vi "TCP- Client.vi"() -> ()   [LabVIEW 2015]
doc: "Demonstrates how to use Network Streams to pass data and commands between two running VIs. This VI passes data to the host VI, based on the frequency specified by the host VI."
panel:
  out "Cluster":cluster{"Frequency":i32}={"Frequency"=10}
  in  "Stop":bool
  in  "Server Closed":string="The server VI closed the connection."
  in  "Client Closed":string="The client VI closed the connection."
  # "Overview: Demonstrates how to use Network Streams to pass data and commands between two running VIs.\nRequirements: Windows\nInstructions:\n1. Run this VI.\n2. Open Simple Network Streams - Host.vi and follow the instructions on its front panel."
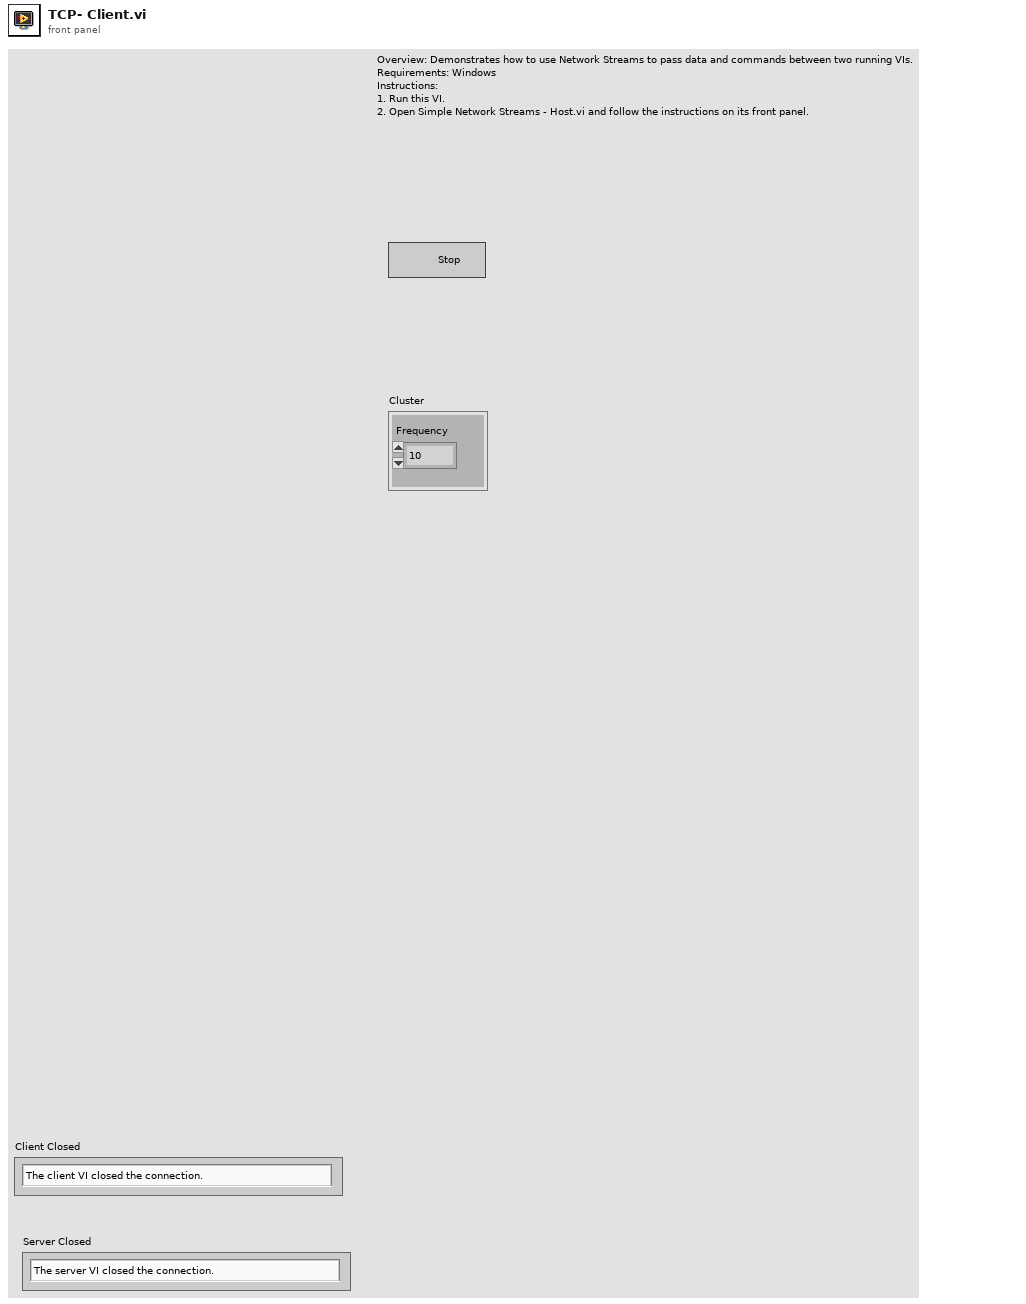
[diagram p1: front panel]
types:
  T1 = cluster{"ID":dbl, "Enable":dbl, "Direction":dbl, "Brake":dbl, "Built-In Encoder":dbl, "Motor Voltage FB":dbl, "Motor Current FB":dbl, "Brake Voltage FB":dbl, "Brake Current FB":dbl, "Up Limit Switch":dbl, "Down Limit Switch":dbl, "Up Limit Config":dbl, "Down Limit Config":dbl, "Motor Current Limit Config":dbl, "Brake Current Limit Config":dbl, "Status":dbl}
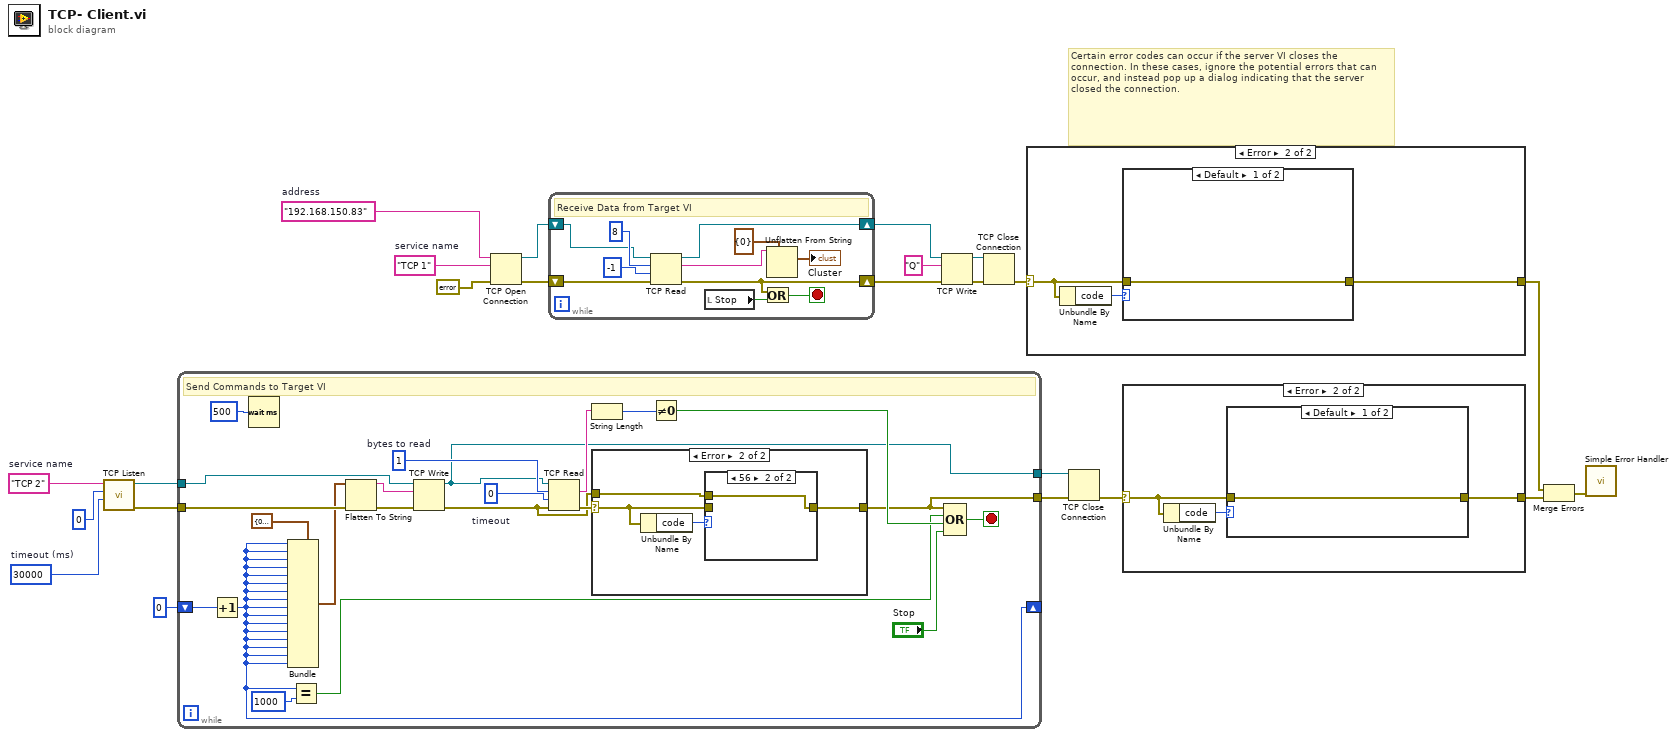
[diagram p0: block diagram]
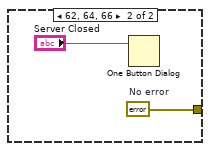
[diagram p3: hidden frame]
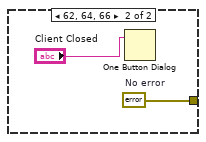
[diagram p5: hidden frame]
diagram:
  w5 = "TCP 1"  # service name
  w17 = "192.168.150.83"  # address
  w6 = "TCP 2"  # service name
  w22 = 30000  # timeout (ms)
  # "Certain error codes can occur if the server VI closes the connection. In these cases, ignore the potential errors that can occur, and instead pop up a dialog indicating that the server closed the connection."
  n1 = call <vilib>:"TCP Listen.vi"("timeout ms (wait forever: -1)"=w22, "port"=u16 0, "service name"=w6) -> ("error out"=w3:errorcluster, "connection ID"=w21:refnum<k5>)  [unwired: 4 in, 3 out]
  n2 = while "Host->Target Command Writer" {
    tunnel: w3 -> [w32]
    tunnel: w21 -> [w45]
    tunnel: [w36] -> w19
    tunnel: [w35] -> w18
    shift-right: [w26] -> _
    shift-left: 0 -> [w29]
    stop <- w38 stop-if-true
    w41 = 0  # timeout
    w40 = 1  # bytes to read
    # "Send Commands to Target VI"
    n3 = Increment(x=w29) -> (x+1=w26:i32)
    n4 = Wait (ms)(milliseconds to wait=u32 500) -> ()  [unwired: 1 out]
    n5 = Bundle(cluster=T1 {"ID"=0.0, "Enable"=0.0, "Direction"=0.0, "Brake"=0.0, "Built-In Encoder"=0.0, "Motor Voltage FB"=0.0, "Motor Current FB"=0.0, "Brake Voltage FB"=0.0, "Brake Current FB"=0.0, "Up Limit Switch"=0.0, "Down Limit Switch"=0.0, "Up Limit Config"=0.0, "Down Limit Config"=0.0, "Motor Current Limit Config"=0.0, "Brake Current Limit Config"=0.0, "Status"=0.0} ("MirrorCoverMotor"), "ID"=w26, "Enable"=w26, "Direction"=w26, "Brake"=w26, "Built-In Encoder"=w26, "Motor Voltage FB"=w26, "Motor Current FB"=w26, "Brake Voltage FB"=w26, "Brake Current FB"=w26, "Up Limit Switch"=w26, "Down Limit Switch"=w26, "Up Limit Config"=w26, "Down Limit Config"=w26, "Motor Current Limit Config"=w26, "Brake Current Limit Config"=w26, "Status"=w26) -> (w30:T1)
    n6 = Equal?(x=w26, y=1000) -> (x = y?=w27:bool)
    n7 = Flatten To String(anything=w30, error in (no error)=w32) -> (data string=w34:string, error out=w33:errorcluster)  [unwired: 2 in, 1 out]
    n8 = TCP Write(connection ID=w45, data in=w34, error in (no error)=w33) -> (connection ID out=w35:refnum<k5>, error out=w39:errorcluster)  [unwired: 2 out]
    n9 = TCP Read(connection ID=w35, bytes to read=w40, error in (no error)=w39, 9:w41) -> (data out=w43:string, error out=w44:errorcluster)  [unwired: 2 out]
    n10 = String Length(string=w43) -> (length=w42:i32)
    n11 = case shown="Error" w44 {
      selector: w44 -> [w46 w49]
      tunnel: [w46 w47] -> w36
      tunnel: w39 -> [_ w48]
      frame No Error {
      }
      frame Error {
        n12 = Unbundle By Name(w49) -> ("code"=w50:i32)
        n13 = case shown="56" w50 {
          tunnel: w49 -> [w51 _]
          tunnel: w48 -> [_ w52]
          tunnel: [w51 w52] -> w47
          frame Default {
          }
          frame 56 {
          }
        }
      }
    }
    n14 = Not Equal To 0?(x=w42) -> (x != 0?=w37:bool)
    n15 = Compound Arithmetic op=OR(w36, w27, w37, "Stop") -> (w38:bool)
  }
  n16 = TCP Open Connection(address=w17, remote port or service name=w5, error in (no error)=errorcluster {"status"=FALSE, "code"=0, "source"=""} ("error out")) -> (connection ID=w16:refnum<k5>, error out=w1:errorcluster)  [unwired: 2 in]
  n17 = while "Target->Host Data Reader" {
    shift-right: [w56] -> w11
    shift-left: w1 -> [w61]
    shift-right: [w60] -> w10
    shift-left: w16 -> [w59]
    stop <- w57 stop-if-true
    # "Receive Data from Target VI"
    n18 = TCP Read(connection ID=w59, bytes to read=8, error in (no error)=w61, 9:-1 ("timeout ms (25000)")) -> (connection ID out=w60:refnum<k5>, data out=w55:string, error out=w56:errorcluster)  [unwired: 1 in]
    n19 = local read "Stop"() -> (w58:bool)
    n20 = Or(x=w56, y=w58) -> (x .or. y?=w57:bool)
    n21 = Unflatten From String(type=cluster{"Frequency":i32} {"Frequency"=0} ("Cluster 2"), binary string=w55) -> (value=→"Cluster":cluster{"Frequency":i32})  [unwired: 3 in, 2 out]
  }
  n22 = TCP Write(connection ID=w10, data in="Q", error in (no error)=w11) -> (connection ID out=w12:refnum<k5>, error out=w13:errorcluster)  [unwired: 2 out]
  n23 = TCP Close Connection(connection ID=w12, error in (no error)=w13) -> (error out=w15:errorcluster)  [unwired: 1 in, 1 out]
  n24 = case shown="Error" w15 {
    selector: w15 -> [w64 w66]
    tunnel: [w64 w65] -> w9
    frame No Error {
    }
    frame Error {
      n25 = Unbundle By Name(w66) -> ("code"=w67:i32)
      n26 = case shown="Default" w67 {
        tunnel: w66 -> [w68 _]
        tunnel: [w68 w70] -> w65
        frame Default {
        }
        frame 62, 64, 66 {
          w70 = errorcluster {"status"=FALSE, "code"=0, "source"=""}  # No error
          n27 = One Button Dialog(message="Server Closed") -> ()  [unwired: 1 in, 1 out]
        }
      }
    }
  }
  n28 = TCP Close Connection(connection ID=w18, error in (no error)=w19) -> (error out=w20:errorcluster)  [unwired: 2 out]
  n29 = case shown="Error" w20 {
    selector: w20 -> [w71 w73]
    tunnel: [w71 w72] -> w8
    frame No Error {
    }
    frame Error {
      n30 = Unbundle By Name(w73) -> ("code"=w74:i32)
      n31 = case shown="Default" w74 {
        tunnel: w73 -> [w75 _]
        tunnel: [w75 w77] -> w72
        frame Default {
        }
        frame 62, 64, 66 {
          w77 = errorcluster {"status"=FALSE, "code"=0, "source"=""}  # No error
          n32 = One Button Dialog(message="Client Closed") -> ()  [unwired: 1 in, 1 out]
        }
      }
    }
  }
  n33 = Merge Errors(w9, w8) -> (w23:errorcluster)
  n34 = call <vilib>:"Simple Error Handler.vi"("error in (no error)"=w23) -> ()  [unwired: 4 in, 5 out]
